vi "Untitled 1.vi"(8 "error in (no error)":errorcluster, 11 "USB-6000 in":refnum<class "USB-6000.lvclass">) -> (0 "error out":errorcluster, 3 "USB-6000 out":refnum<class "USB-6000.lvclass">)   [LabVIEW 2025, in "USB IO.lvlib" / "USB-6000.lvclass"]
uses:
  USB-6000.lvclass
  USB-6000.lvclass/USB-6000.ctl
  <vilib>/DAQmx/write.llb/DAQmx Write (Digital 1D Bool 1Chan 1Samp).vi
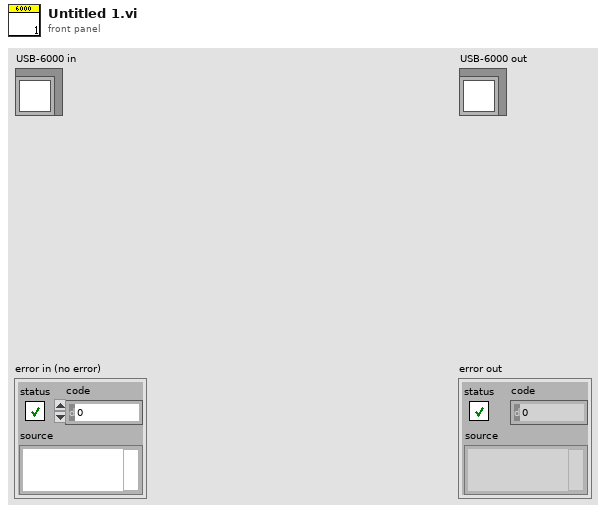
[diagram p1: front panel]
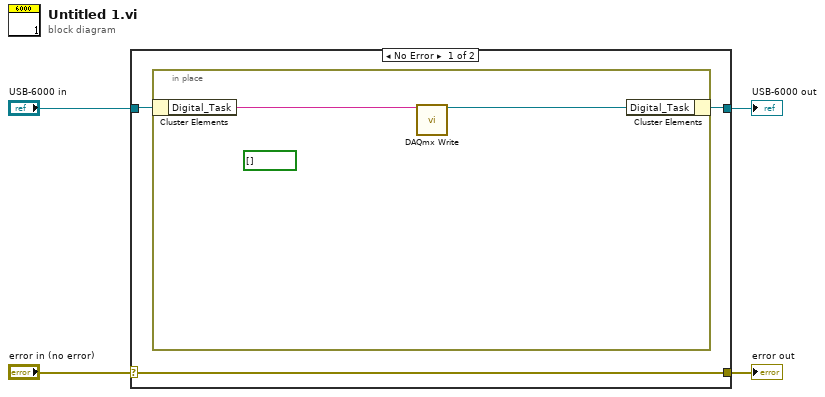
[diagram p0: block diagram]
diagram:
  n1 = case shown="No Error" "error in (no error)" {
    selector: "error in (no error)" -> [w7 w11]
    tunnel: [w7 w11] -> w3
    tunnel: [w5 w10] -> w1
    tunnel: "USB-6000 in" -> [w6 w10]
    frame No Error {
      n2 = in-place {
        (unwired) bool[] [] ("data")
        n3 = in-place-cluster #1(w6) -> ("Digital_Task"=w8:string)
        n4 = call-poly <vilib>:"DAQmx Write.vi"("task/channels in"=w8) -> ("task out"=w9:refnum<k21>)  [unwired: 12 in, 2 out]
        n5 = in-place-cluster #1("Digital_Task"=w9) -> (w5:refnum<class "USB-6000.lvclass">)
      }
    }
    frame Error {
    }
  }
  "error out" <- w3
  "USB-6000 out" <- w1
